vi "CRYDataView Socket Log.vi"(9 "sOption":string, 10 "Graph Number":i32) -> (3 "sOption Out":string)   [LabVIEW 2013]
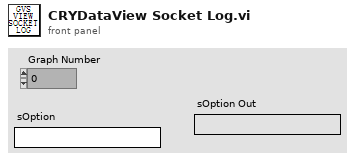
[diagram p1: front panel]
types:
  T1 = enum16{"open", "replace", "create", "open or create", "replace or create", "replace or create with confirmation"}
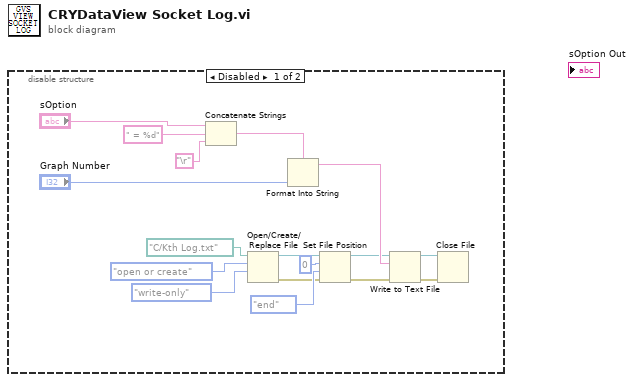
[diagram p0: block diagram]
diagram:
  n1 = disable-structure shown="Disabled" {
    frame Disabled {
      n2 = Concatenate Strings("sOption", " = %d" ("string"), "\r") -> (w1:string)
      n3 = Open/Create/Replace File(file path (use dialog)=path "C:/Kth Log.txt", operation (0:open)=T1."open or create", access (0:read/write)=enum16{"read/write", "read-only", "write-only"}."write-only") -> (refnum out=w9:refnum<file>, error out=w5:errorcluster)  [unwired: 3 in, 1 out]
      n4 = Format Into String(format string=w1, "Graph Number") -> (resulting string=w13:string)  [unwired: 2 in, 1 out]
      n5 = Set File Position(offset (in bytes) (0)=i64 0, refnum=w9, from (0:start)=enum16{"start", "end", "current"}."end", error in=w5) -> (refnum out=w7:refnum<file>, error out=w4:errorcluster)
      n6 = Write to Text File(file (use dialog)=w7, text=w13, error in=w4) -> (refnum out=w11:refnum<file>, error out=w12:errorcluster)  [unwired: 1 in, 1 out]
      n7 = Close File(refnum=w11, error in=w12) -> ()  [unwired: 2 out]
    }
    frame Enabled {
    }
  }
